vi "mWmotor_Main_calib.vi"() -> ()   [LabVIEW 2019]
uses:
  SubVI/Automatic mode/Controller decision.ctl
  SubVI/Motor Controller/Motor Class/Motor.lvclass
  SubVI/Beam/Beam.lvclass
  SubVI/Automation/Automation.lvclass
  SubVI/Simulation/Signaller/Signaller.lvclass
panel:
  out "Intensity Found":bool
  out "Last spill Intensity \n(protons)":dbl format="%#_6e"
  in  "Reset the counter":bool
  in  "Pause  accumulation":bool
  out "Spil Counter":dbl
  out "Accumulated Intensity (protons)":dbl format="%#_6e"
  out "Spill ID":dbl format="%#_6f"
  out "Current Frequencuy  (GHz)\n(Mapped)":dbl format="%_6g"
  out "EIP Frequency (GHz)":dbl format="%#_7g"
  out "Current possition (rev)":dbl
  in  "Move to frequecy":bool
  in  "Set possition (rev)":dbl=0.36 min=0.0 max=4.1
  in  "Degrees":dbl=0.36 min=0.36
  in  "CCW":bool
  in  "CW":bool
  in  "stop motor":bool
  in  "Set Freq (GHz)":dbl=140.0 min=140.0 max=141.9
  out "Upper (GHz)":dbl
  out "Lower (GHz)":dbl
  in  "Range(MHz)":dbl=10.0
  in  "Center Frequency(GHz)":dbl=140.2
  in  "Seek Function":enum16{"Rate based", "Ploarization(avg) based"}(ring)
  out "Motor Action":T1
  out "Has all samples":bool
  in  "Automatic step size (rev)":dbl=0.001
  in  "Seek type":enum32{"Seek Positive", "Seek Negative"}(radio)
  in  "Start Auto control":bool
  in  "Bypass Freq check":bool
  out "Gradients":dbl[](array[numeric])
  out "Recovery sequence":string
  in  "Recovery loop stop":bool
  in  "Recovery":bool
  out "Temp alarms":bool
  in  "Start Recovery":bool
  in  "Record Data":bool=TRUE
  in  "Warning Sound":bool
  out "EIO Temp":string
  out "chart_temp 2":waveform(dbl)[](graph)=[{"t0"=timestamp(3772890114.31303 s since 1904-01-01), "dt"=1.0, "Y"=[0.8687935985565186]}, {"t0"=timestamp(3772890114.31303 s since 1904-01-01), "dt"=1.0, "Y"=[86.87935985565186]}, {"t0"=timestamp(3772890114.31303 s since 1904-01-01), "dt"=1.0, "Y"=[30.48853325313992]}, {"t0"=timestamp(3772890114.31303 s since 1904-01-01), "dt"=1.0, "Y"=[303.6385332531399]}] caption="EIO temperatures"
  out "T_array":dbl[](array[numeric])
  out "Accumilated dose":waveform(dbl)[](graph)=[{"t0"=timestamp(3772890114.31303 s since 1904-01-01), "dt"=1.0, "Y"=[0.8687935985565186]}, {"t0"=timestamp(3772890114.31303 s since 1904-01-01), "dt"=1.0, "Y"=[86.87935985565186]}, {"t0"=timestamp(3772890114.31303 s since 1904-01-01), "dt"=1.0, "Y"=[30.48853325313992]}, {"t0"=timestamp(3772890114.31303 s since 1904-01-01), "dt"=1.0, "Y"=[303.6385332531399]}]
  out "Calibration run flag":bool
  out "New data point":bool
  out "EIPFRQ":waveform(dbl)[](graph)=[{"t0"=timestamp(3772890114.31303 s since 1904-01-01), "dt"=1.0, "Y"=[0.8687935985565186]}, {"t0"=timestamp(3772890114.31303 s since 1904-01-01), "dt"=1.0, "Y"=[86.87935985565186]}, {"t0"=timestamp(3772890114.31303 s since 1904-01-01), "dt"=1.0, "Y"=[30.48853325313992]}, {"t0"=timestamp(3772890114.31303 s since 1904-01-01), "dt"=1.0, "Y"=[303.6385332531399]}]
  out "Simulated Eventnum":i64
  out "Simulated polarization":dbl
  in  "Launch simulation":bool
  in  "Polarization data source":enum32{"NMR", "SIM"}(radio)
  out "EIO Temp reading":bool
  out "Motor alarm":bool
  out "NMR data issue":bool
  out "Loop Running":bool
  in  "NMR IP":string="192.168.24.191"
  in  "EIP":refnum<visa-resource-name>="GPIB0::5::INSTR"
  in  "ADC Port":refnum<visa-resource-name>="COM4"
  in  "stop VI":bool
  in  "Motor Port":refnum<visa-resource-name>="COM3"
  out "Current motor possition (Revolutions)":dbl(knob) caption="Current Angle" scale=0.0..4.1
  out "CCW":bool caption="CCW Limit"
  out "CW":bool caption="CW Limit"
  out "ADC Count":i32(slide) scale=0.0..32768.0
  out "ADC Count":i32
  out "Motor Running":bool
  out "Polarization":dbl format="%#_3f"
  out "Eventnum":i64
  out "Polarization Chart":waveform(dbl)[](graph)=[{"t0"=timestamp(3772890114.31303 s since 1904-01-01), "dt"=1.0, "Y"=[0.8687935985565186]}, {"t0"=timestamp(3772890114.31303 s since 1904-01-01), "dt"=1.0, "Y"=[86.87935985565186]}, {"t0"=timestamp(3772890114.31303 s since 1904-01-01), "dt"=1.0, "Y"=[30.48853325313992]}, {"t0"=timestamp(3772890114.31303 s since 1904-01-01), "dt"=1.0, "Y"=[303.6385332531399]}]
  in  "Calibration panel":bool
  in  "Calibration panel":enum32{"Page 1", "Page 2"}(tab)
  out "Lower Frequency":dbl
  out "Lower  possition":dbl
  in  "R_lower":bool
  out "New Intercept":dbl=138.611
  out "New Slope":dbl=0.864
  in  "Use_para":bool
  out "Upper  possition":dbl
  in  "cal_para":bool
  out "Upper Frequecy":dbl
  in  "R_upper":bool
  out "Intercept":dbl
  out "Slope":dbl
  in  "Set_motor":bool
  in  "File Path Control":path=path "C:/Users/ptgroup/Desktop/github/Microwave-motor-control/config.ini"
  out "Speed  (rev/s)":dbl
  in  "File Name":string
  out "Frequency (GHz)":dbl
  out "Possition (Rev)":dbl format="%_4g"
  out "New data  saved":bool
  out "Recording":bool
  in  "Stop calibration":bool
  in  "Move direction":enum32{"CCW", "CW"}(radio)
  in  "Start calibration":bool
  in  "Step size (rev)":dbl
  out "Estimated Possition":dbl
  out "error out":errorcluster
  # "Warnings"
  # "Manual Motor Control"
  # "Beam information"
  # "Auto control   Setup"
  # "Auto control   Parameters"
  # "Communication  Setup"
  # "Current motor possition (Rev)"
  # "Calibration Panel"
  # "Calibration panel"
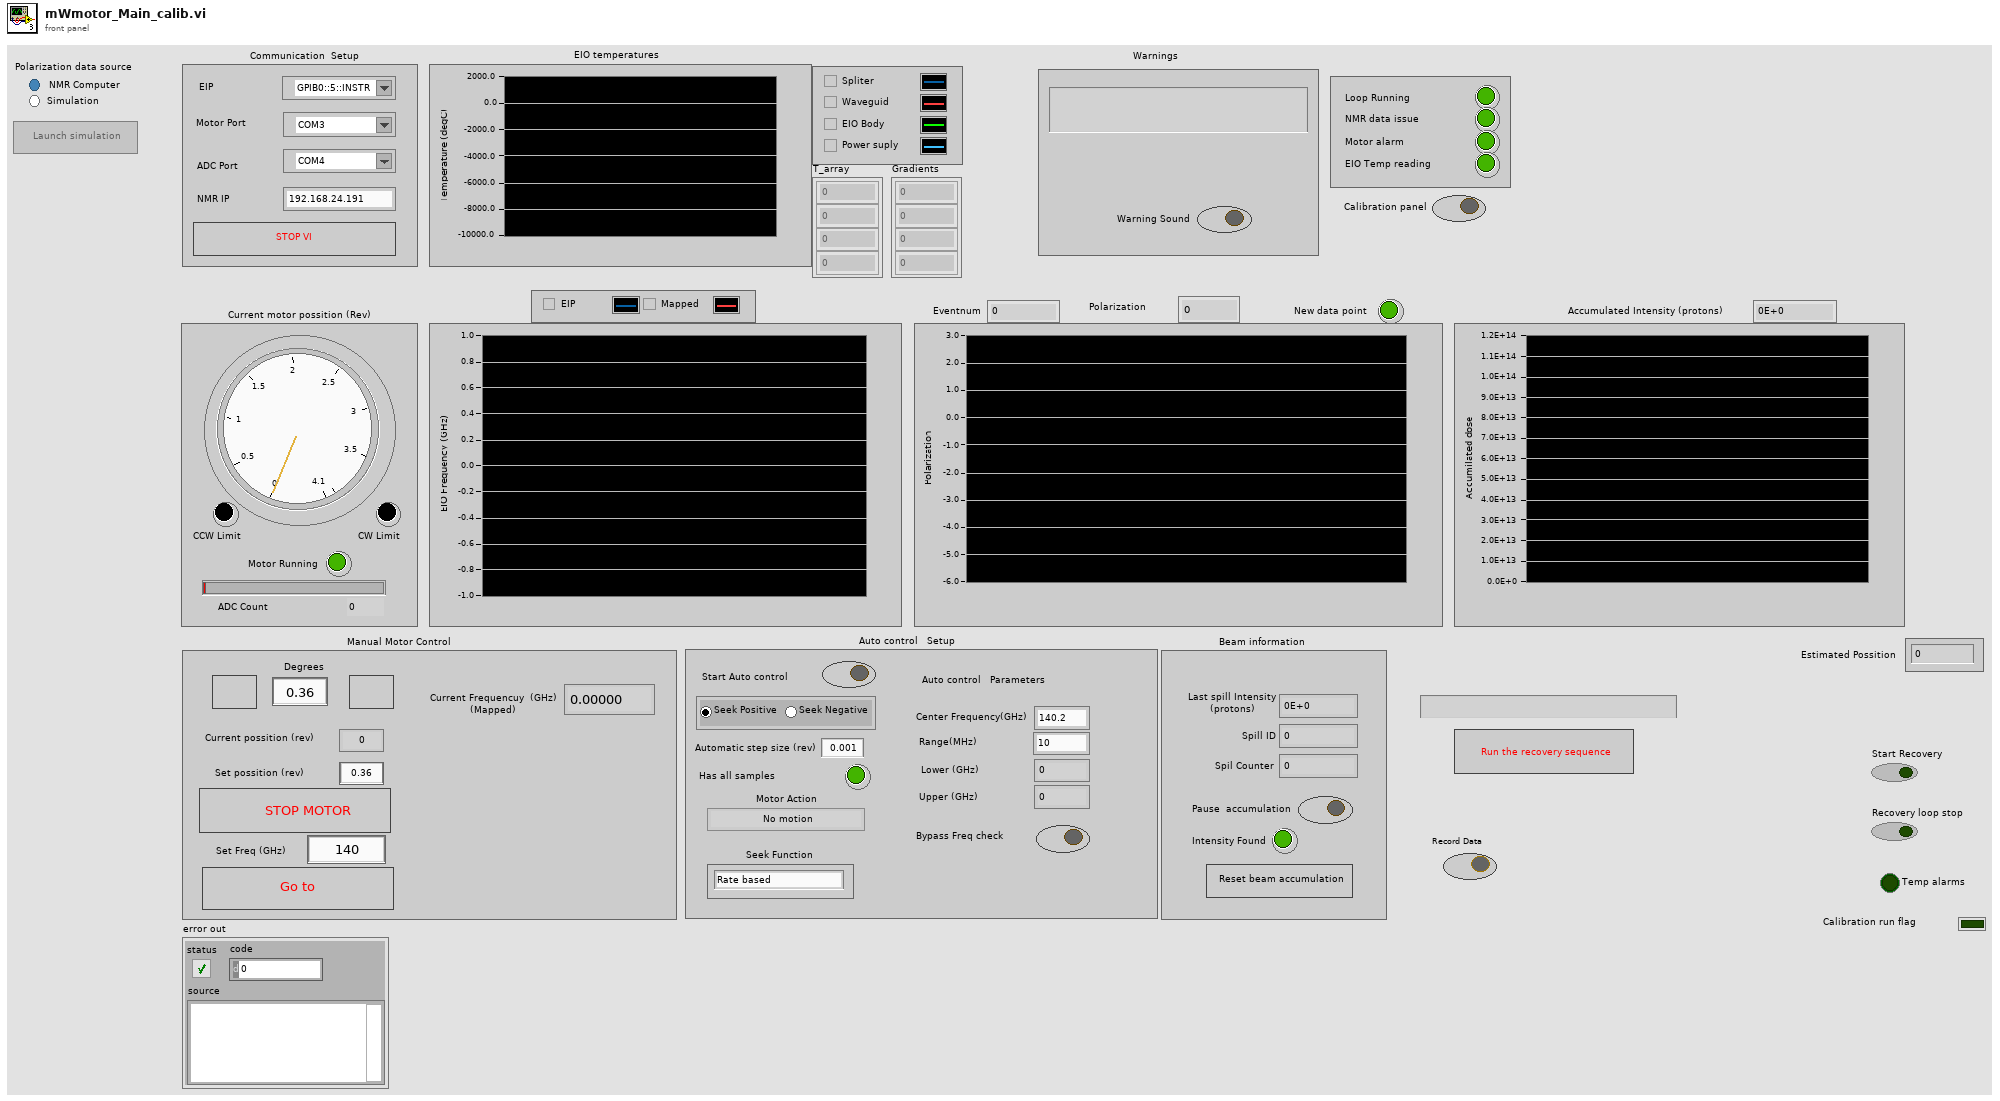
[diagram p1: front panel]
types:
  T1 = typedef "Controller decision.ctl" = enum16{"No motion", "Switch direction", "Keep current direction"}
  T2 = enum8{"Enabled", "Disabled", "Disabled and Grayed Out"}
  T3 = typedef "Sound Output Task ID.ctl" = u32
  T4 = enum32{"Bad", "Idle", "Run top level", "Running"}
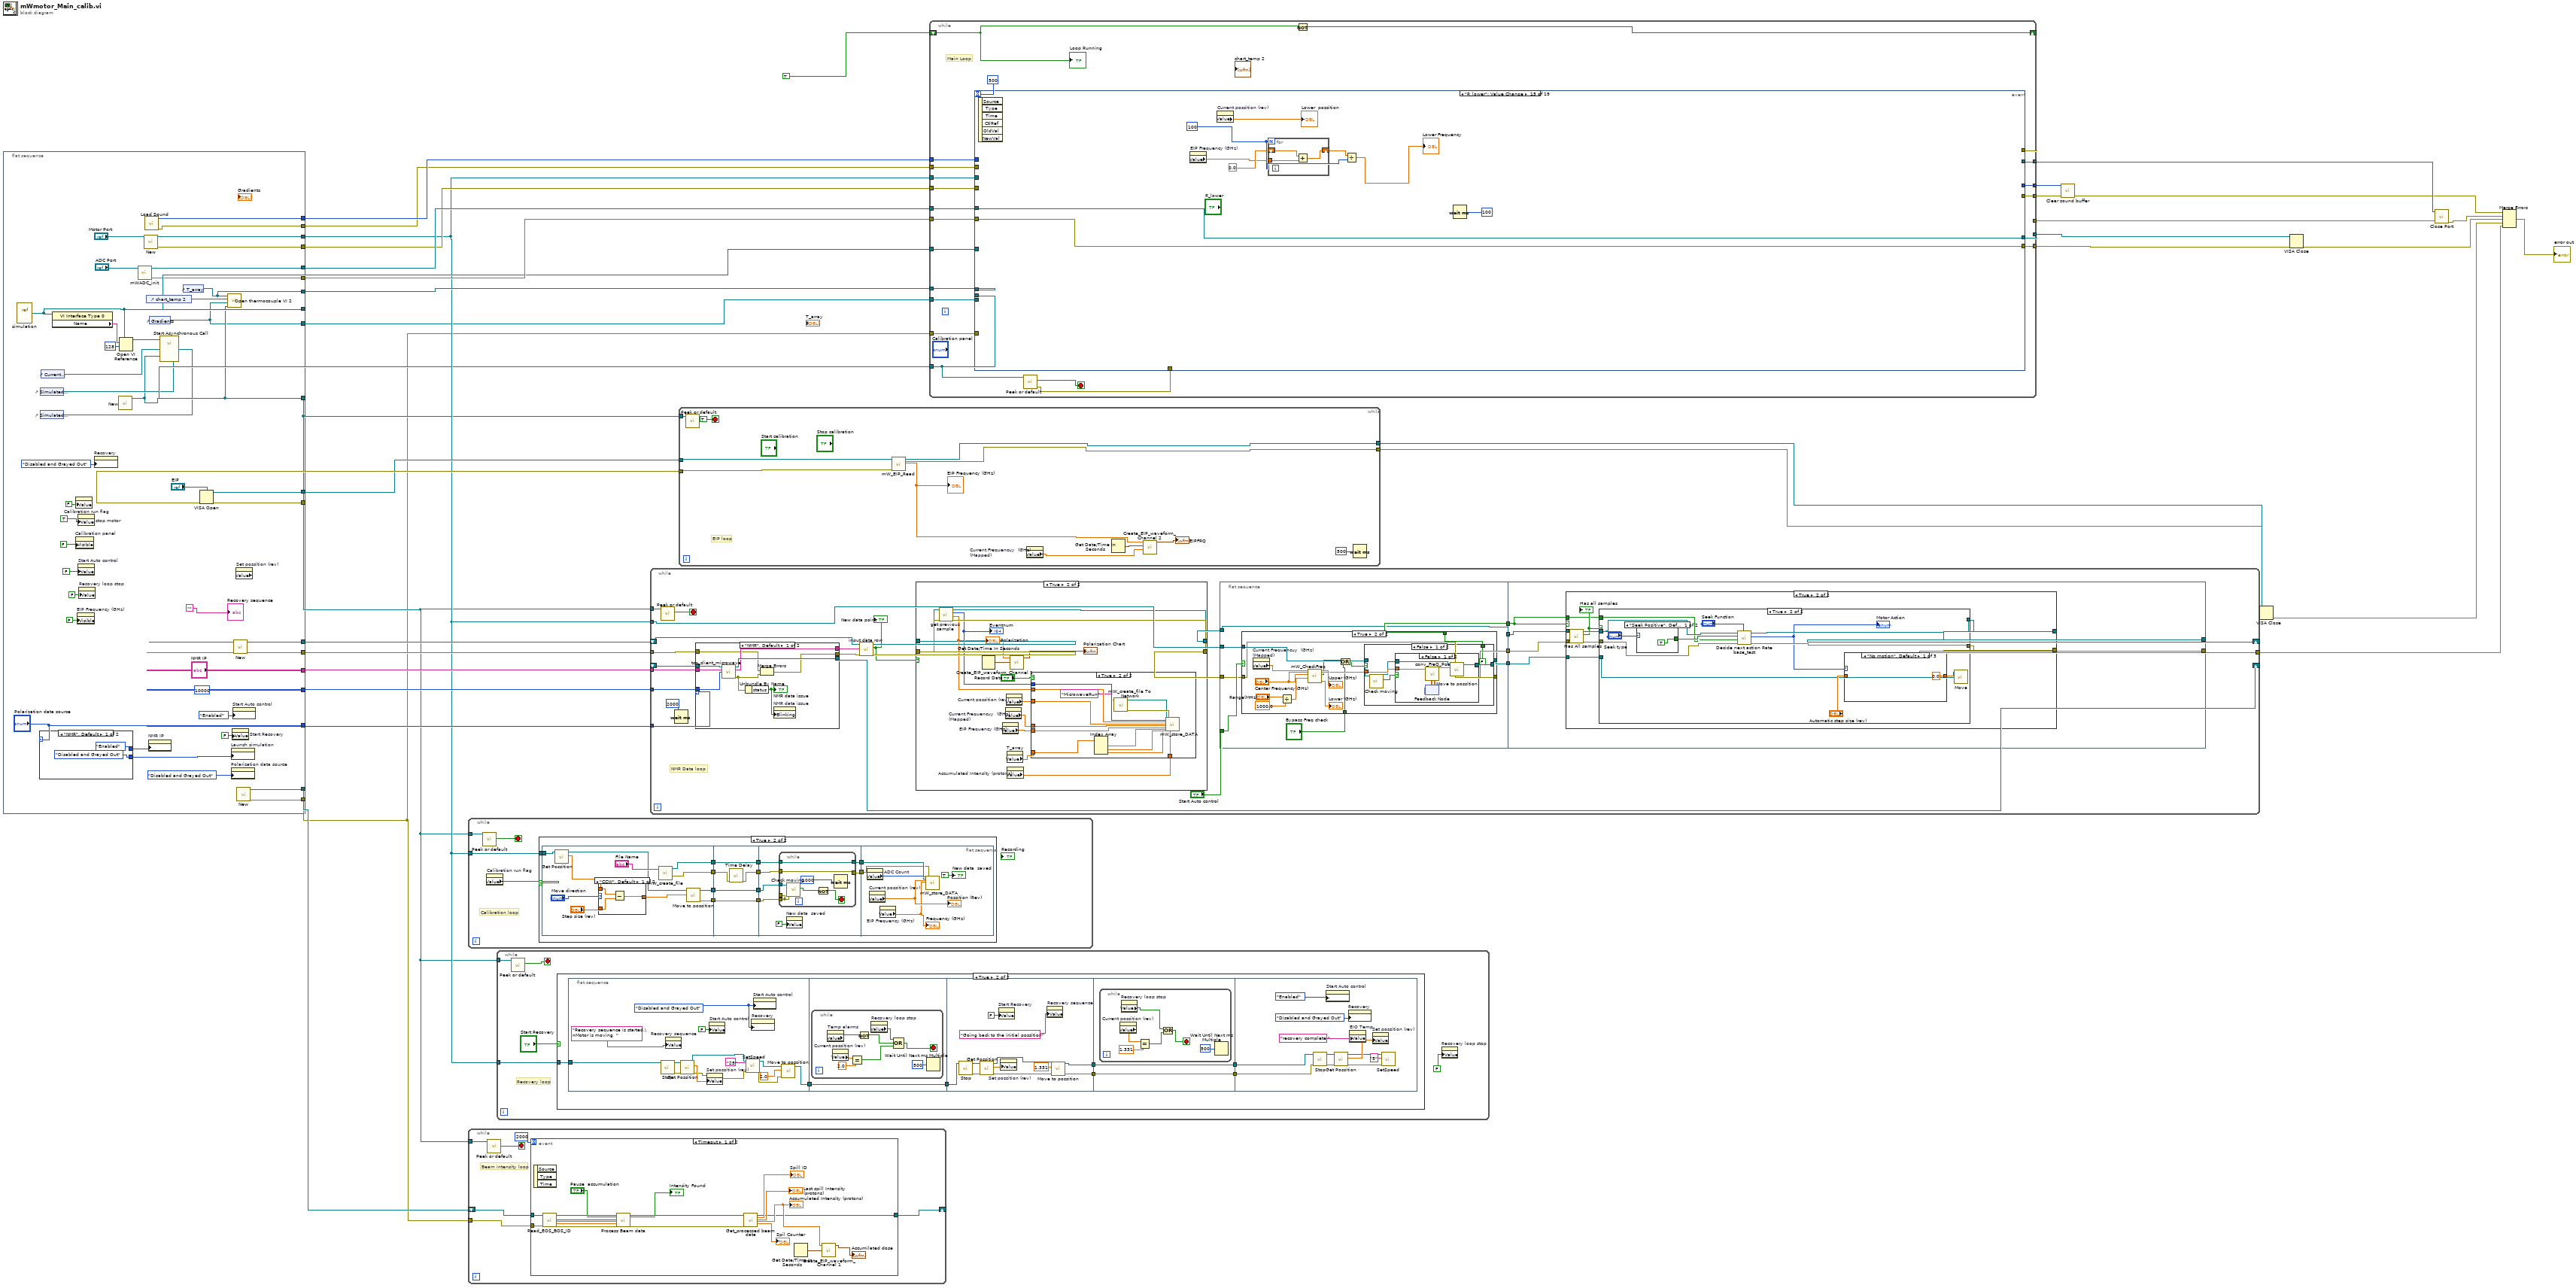
[diagram p0: block diagram]
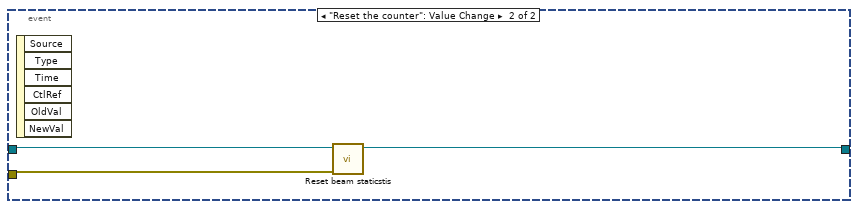
[diagram p2: hidden frame]
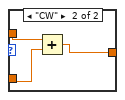
[diagram p5: hidden frame]
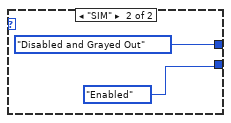
[diagram p6: hidden frame]
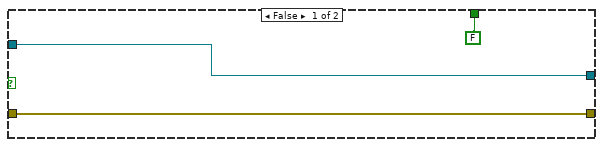
[diagram p7: hidden frame]
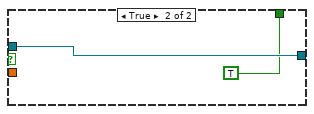
[diagram p9: hidden frame]
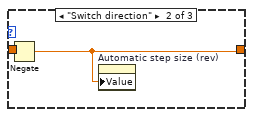
[diagram p12: hidden frame]
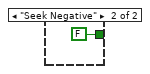
[diagram p14: hidden frame]
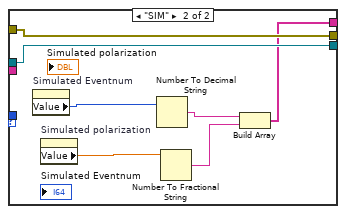
[diagram p17: hidden frame]
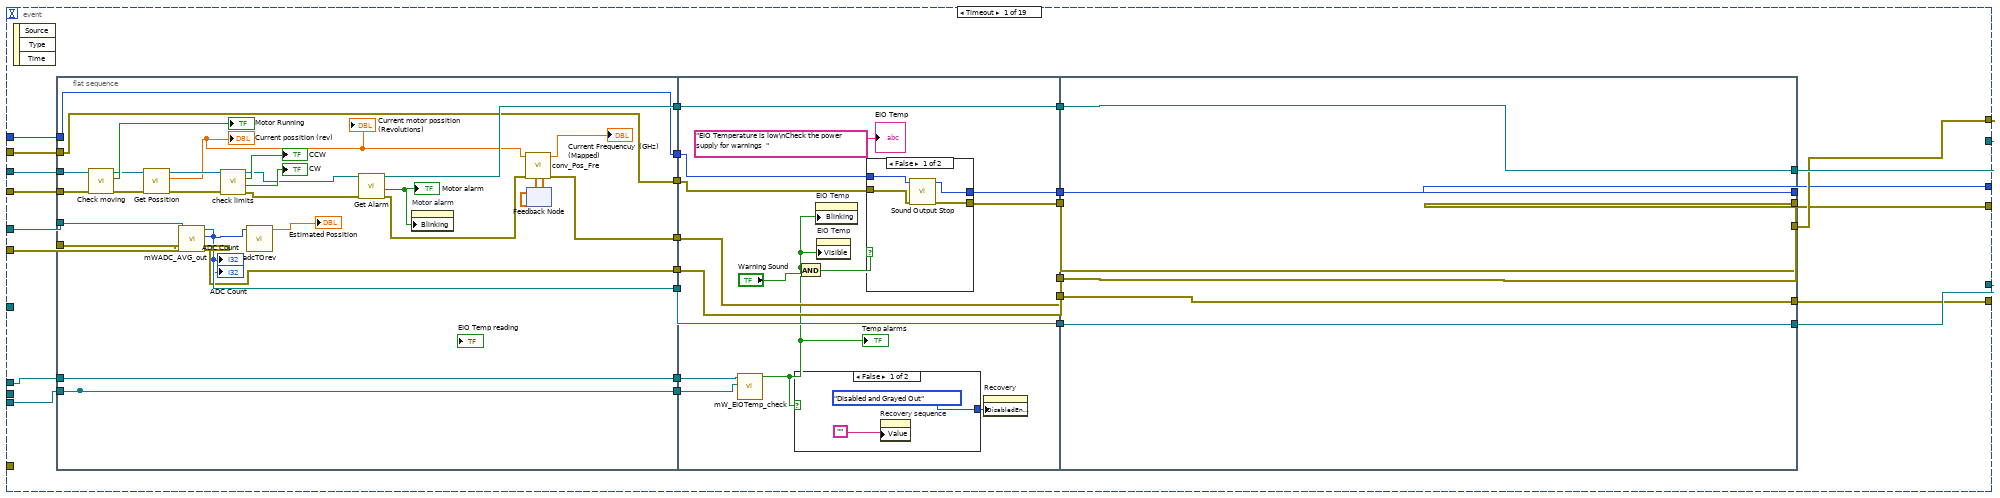
[diagram p18: hidden frame]
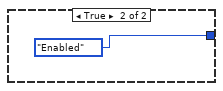
[diagram p19: hidden frame]
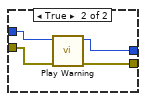
[diagram p20: hidden frame]
diagram:
  n1 = flat-sequence {
    tunnel: [w75] -> w33
    tunnel: [w74] -> w30
    tunnel: [w73] -> w27
    tunnel: [w72] -> w26
    tunnel: [w68] -> w5
    tunnel: [w67] -> w23
    tunnel: [u16 10000 ("port")] -> w18
    tunnel: [w65] -> w17
    tunnel: [w64] -> w16
    tunnel: ["NMR IP"] -> w15
    tunnel: [w60] -> w13
    tunnel: [w47] -> w3
    tunnel: ["Polarization data source"] -> w12
    tunnel: [w46] -> w11
    tunnel: [w45] -> w10
    tunnel: [w44] -> w9
    tunnel: [w38] -> w4
    tunnel: [w37] -> w2
    tunnel: [w36] -> w1
    frame #0 {
      n2 = vi-ref "simulation.vi"() -> (w60:refnum<vi>)
      n3 = case shown="\"NMR\", Default" "Polarization data source" {
        tunnel: [T2."Disabled and Grayed Out" ("Disabled") T2."Enabled" ("Disabled")] -> w54
        tunnel: [T2."Enabled" ("Disabled") T2."Disabled and Grayed Out" ("Disabled")] -> w52
        frame "NMR", Default {
        }
        frame "SIM" {
        }
      }
      n4 = control-ref of="Simulated Eventnum"() -> (w56:refnum<vi>)
      n5 = control-ref of="Simulated polarization"() -> (w57:refnum<vi>)
      n6 = control-ref of="Current Frequencuy  (GHz)\n(Mapped)"() -> (w58:refnum<vi>)
      n7 = property class="VI Interface Type 0"(reference=w60) -> ("Name"=w62:string)  [unwired: 1 in, 2 out]
      n8 = property on="Calibration panel" class="TabCtl (strict)"("Visible"=FALSE) -> ()  [unwired: 2 in, 2 out]
      n9 = property on="Calibration run flag" class="Bool (strict)"("Value"=FALSE ("Calibration run flag")) -> ()  [unwired: 2 in, 2 out]
      n10 = property on="EIP Frequency (GHz)" class="DigNum (strict)"("Visible"=FALSE) -> ()  [unwired: 2 in, 2 out]
      n11 = property on="stop motor" class="Bool (strict)"("Value"=TRUE ("Value (Signaling)")) -> ()  [unwired: 2 in, 2 out]
      n12 = property on="Start Auto control" class="Bool (strict)"("Value"=FALSE ("Start Auto control")) -> ()  [unwired: 2 in, 2 out]
      n13 = property on="Recovery loop stop" class="Bool (strict)"("Value"=FALSE ("Recovery loop stop")) -> ()  [unwired: 2 in, 2 out]
      n14 = property on="Recovery" class="Bool (strict)"("DisabledEnum"=T2."Disabled and Grayed Out" ("Disabled")) -> ()  [unwired: 2 in, 2 out]
      n15 = call "New.vi"() -> ("Signaller out"=w47:refnum<class "Signaller.lvclass">)  [unwired: 11 in]
      n16 = Open VI Reference(type specifier VI Refnum (for type only)=w60, vi path=w62, options=128) -> (vi reference=w59:refnum<vi>)  [unwired: 3 in, 1 out]
      n17 = call "mWADC_init.vi"("mWADC_Port"="ADC Port") -> ("error out"=w74:errorcluster, "reference out"=w75:refnum<visa-resource-name>)  [unwired: 9 in]
      n18 = call "New.vi"("VISA resource name"="Motor Port") -> ("error out"=w67:errorcluster, "Motor out"=w68:refnum<class "Motor.lvclass">)  [unwired: 9 in]
      n19 = call "Load Sound.vi"() -> ("error out"=w44:errorcluster, "task ID out"=w45:T3)  [unwired: 10 in]
      n20 = control-ref of="chart_temp 2"() -> (w48:refnum<vi>)
      n21 = property on="NMR IP" class="Str"("DisabledEnum"=w52) -> ()  [unwired: 2 in, 2 out]
      n22 = control-ref of="Gradients"() -> (w38:refnum<vi>)
      n23 = call-by-ref "Start Asynchronous Call"(reference=w59, "Eventnum refnum"=w56, "Polarization refnum"=w57, "Stop signaller"=w47, "Frequency refnum"=w58) -> ()  [unwired: 1 in, 2 out]
      n24 = control-ref of="T_array"() -> (w46:refnum<vi>)
      n25 = VISA Open(VISA resource name="EIP") -> (VISA resource name=w72:refnum<visa-resource-name>, error out=w73:errorcluster)  [unwired: 4 in]
      n26 = call "Open thermocouple VI 2.vi"("Signaller in"=w47, "Gradients"=w38, "chart_temp ref"=w48, "Temperaturs"=w46) -> ()  [unwired: 8 in]
      n27 = property on="Launch simulation" class="Bool"("DisabledEnum"=w54) -> ()  [unwired: 2 in, 2 out]
      n28 = property on="Polarization data source" class="RadioBtnsControl (strict)"("DisabledEnum"=T2."Disabled and Grayed Out" ("Disabled")) -> ()  [unwired: 2 in, 2 out]
      n29 = property on="Start Recovery" class="Bool (strict)"("Value"=FALSE ("Start Recovery")) -> ()  [unwired: 2 in, 2 out]
      n30 = property on="Start Auto control" class="Bool (strict)"("DisabledEnum"=T2."Enabled" ("Disabled")) -> ()  [unwired: 2 in, 2 out]
      n31 = call "New.vi"() -> ("error out"=w64:errorcluster, "Automation out"=w65:refnum<class "Automation.lvclass">)  [unwired: 10 in]
      n32 = property on="Set possition (rev)" class="DigNum (strict)" props=["Value"]() -> ()  [unwired: 2 in, 3 out]
      n33 = call "New.vi"() -> ("error out"=w36:errorcluster, "Beam out"=w37:refnum<class "Beam.lvclass">)  [unwired: 10 in]
      "Recovery sequence" <- ""
    }
  }
  n34 = while {
    tunnel: w3 -> [w84]
    tunnel: w5 -> [w82]
    stop <- w81 stop-if-true
    # "Calibration loop"
    n35 = call "Peek or default.vi"("Signaller in"=w84) -> ("Has signal?"=w81:bool)  [unwired: 8 in, 2 out]
    n36 = property on="Calibration run flag" class="Bool (strict)"() -> ("Value"=w83:bool)  [unwired: 2 in, 2 out]
    n37 = case shown="True" w83 {
      tunnel: w82 -> [_ w89]
      frame False {
      }
      frame True {
        n38 = flat-sequence {
          tunnel: [w106] -> w93
          tunnel: [w105] -> w91
          tunnel: w89 -> [w100]
          tunnel: [w97] -> w88
          tunnel: [w96] -> w85
          tunnel: w93 -> [w116]
          tunnel: [w115] -> w92
          tunnel: w91 -> [w117]
          tunnel: [w117] -> w90
          tunnel: w88 -> [w114]
          tunnel: [w114] -> w87
          tunnel: [w113] -> w86
          tunnel: w85 -> [w113]
          tunnel: [w123] -> w95
          tunnel: w92 -> [w124]
          tunnel: w90 -> [w121]
          tunnel: [w122] -> w94
          tunnel: w87 -> [w119]
          tunnel: w86 -> [w120]
          tunnel: w95 -> [w132]
          tunnel: w94 -> [w136]
          frame #0 {
            n39 = call "Get Possition.vi"("Motor in"=w100) -> ("Revolutions"=w101:dbl, "Motor out"=w98:refnum<class "Motor.lvclass">)  [unwired: 8 in, 1 out]
            n40 = case shown="\"CCW\", Default" "Move direction" {
              tunnel: [w107 w112] -> w99
              tunnel: "Step size (rev)" -> [w108 w111]
              tunnel: w101 -> [w109 w110]
              frame "CCW", Default {
                n41 = Subtract(x=w109, y=w108) -> (x-y=w107:dbl)
              }
              frame "CW" {
                n42 = Add(x=w110, y=w111) -> (x+y=w112:dbl)
              }
            }
            n43 = call "mW_create_file.vi"("File Name"="File Name") -> ("error out"=w106:errorcluster, "dup path"=w105:path)  [unwired: 9 in]
            n44 = call "Move to possition.vi"("absolute possition(rev)"=w99, "Motor in"=w98) -> ("error out"=w97:errorcluster, "Motor out"=w96:refnum<class "Motor.lvclass">)  [unwired: 8 in]
          }
          frame #1 {
            n45 = call "Time Delay"("error in (no error)"=w116) -> ("error out"=w115:errorcluster)  [unwired: 10 in]
          }
          frame #2 {
            n46 = while {
              tunnel: [w130] -> w123
              tunnel: w124 -> [w130]
              tunnel: [w129] -> w122
              tunnel: w121 -> [w129]
              tunnel: w120 -> [w127]
              tunnel: w119 -> [w125]
              tunnel: [w125] -> _
              stop <- w131 stop-if-true
              n47 = call "Check moving.vi"("error in (no error)"=w125, "Motor in"=w127) -> ("IS Move"=w128:bool)  [unwired: 7 in, 2 out]
              n48 = Not(x=w128) -> (.not. x?=w131:bool)
              n49 = Wait (ms)(milliseconds to wait=u32 1000) -> ()  [unwired: 1 out]
            }
            n50 = property on="New data  saved" class="Bool (strict)"("Value"=FALSE ("New data  saved")) -> ()  [unwired: 2 in, 2 out]
          }
          frame #3 {
            n51 = property on="ADC Count" class="DigNum (strict)"() -> ("Value"=w135:i32)  [unwired: 2 in, 2 out]
            n52 = property on="Current possition (rev)" class="DigNum (strict)"() -> ("Value"=w134:dbl)  [unwired: 2 in, 2 out]
            "Possition (Rev)" <- w134
            n53 = property on="EIP Frequency (GHz)" class="DigNum (strict)"() -> ("Value"=w133:dbl)  [unwired: 2 in, 2 out]
            "Frequency (GHz)" <- w133
            n54 = call "mW_store_DATA.vi"("file path (dialog if empty)"=w136, "col1"=w135, "col2"=w134, "col3"=w133, "error in (no error)"=w132) -> ()  [unwired: 22 in, 1 out]
            "New data  saved" <- TRUE ("New data  saved")
          }
        }
      }
    }
  }
  n55 = while {
    tunnel: w3 -> [w143]
    tunnel: w1 -> [w141]
    shift-right: [w140] -> _
    shift-left: w2 -> [w142]
    stop <- w138 stop-if-true
    # "Beam intensity loop"
    n56 = call "Peek or default.vi"("Signaller in"=w143) -> ("Has signal?"=w138:bool)  [unwired: 8 in, 2 out]
    n57 = event shown="[0] Timeout" {
      selector: _ -> [_ _]
      dyn-events: _ -> [_ _]
      timeout: 2000 -> [_ _]
      tunnel: w142 -> [w161 w164]
      tunnel: w141 -> [w160 w163]
      tunnel: [w153 w162] -> w140
      event Timeout {
        n58 = event-data() -> ()  [unwired: 1 in, 3 out]
        n59 = call-dynamic "Read_EOS_BOS_ID.vi"("Beam in"=w161, "error in (no error)"=w160) -> ("Beam out"=w147:refnum<class "Beam.lvclass">, "Spill ID"=w150:i32, "BOS Time"=w149:dbl, "EOS Time"=w148:dbl, "error out"=w152:errorcluster)  [unwired: 8 in, 1 out]
        n60 = call "Process Beam data.vi"("Beam in"=w147, "Pause"="Pause  accumulation", "Spill ID"=w150, "BOS"=w149, "EOS"=w148, "error in (no error)"=w152) -> ("Beam out"=w146:refnum<class "Beam.lvclass">, "Intensity Found"=→"Intensity Found":bool, "error out"=w151:errorcluster)  [unwired: 11 in]
        n61 = call "Get_processed beam data.vi"("Beam in"=w146, "error in (no error)"=w151) -> ("Beam out"=w153:refnum<class "Beam.lvclass">, "Spill ID"=→"Spill ID":dbl, "Recent spill Intensity"=→"Last spill Intensity \n(protons)":dbl, "Acumilated Intensity"=w156:dbl, "Spil Counter"=→"Spil Counter":dbl)  [unwired: 12 in, 1 out]
        "Accumulated Intensity (protons)" <- w156
        n62 = Get Date/Time In Seconds() -> (seconds since 1Jan1904=w157:timestamp)
        n63 = call "Create_EIP_waveform_Channel 1.vi"("time"=w157, "Channel 1"=w156) -> ("waveform_array"=→"Accumilated dose":waveform(dbl)[])  [unwired: 9 in]
      }
      event "Reset the counter": Value Change {
        n64 = event-data() -> ()  [unwired: 1 in, 6 out]
        n65 = call "Reset beam staticstis.vi"("error in (no error)"=w163, "Beam in"=w164) -> ("Beam out"=w162:refnum<class "Beam.lvclass">)  [unwired: 8 in, 1 out]
      }
    }
  }
  n66 = while {
    tunnel: w3 -> [w169]
    tunnel: w5 -> [w167]
    stop <- w165 stop-if-true
    # "Recovery loop"
    n67 = call "Peek or default.vi"("Signaller in"=w169) -> ("Has signal?"=w165:bool)  [unwired: 8 in, 2 out]
    n68 = case shown="True" "Start Recovery" {
      tunnel: w167 -> [_ w176]
      frame False {
      }
      frame True {
        n69 = flat-sequence {
          tunnel: w176 -> [w187]
          tunnel: [w184] -> w175
          tunnel: w175 -> [w192]
          tunnel: [w192] -> w174
          tunnel: w174 -> [w209]
          tunnel: [w203] -> w172
          tunnel: [w202] -> w170
          tunnel: [w213] -> w173
          tunnel: w172 -> [w213]
          tunnel: [w212] -> w171
          tunnel: w170 -> [w212]
          tunnel: w173 -> [w227]
          tunnel: w171 -> [w226]
          frame #0 {
            w182 = T2."Disabled and Grayed Out" ("Disabled")
            n70 = call "Stop.vi"("Motor in"=w187) -> ("error out"=w190:errorcluster, "Motor out"=w189:refnum<class "Motor.lvclass">)  [unwired: 9 in]
            n71 = property on="Recovery sequence" class="Str"("Value"="Recovery sequence is started.\nMotor is moving  " ("EIO Temp")) -> ()  [unwired: 2 in, 2 out]
            n72 = call "Get Possition.vi"("error in (no error)"=w190, "Motor in"=w189) -> ("error out"=w185:errorcluster, "Revolutions"=w188:dbl, "Motor out"=w181:refnum<class "Motor.lvclass">)  [unwired: 7 in]
            n73 = property on="Set possition (rev)" class="DigNum (strict)"(error in=w185, "Value"=w188) -> (error out=w179:errorcluster)  [unwired: 1 in, 1 out]
            n74 = property on="Start Auto control" class="Bool (strict)"("Value"=FALSE ("Start Auto control")) -> ()  [unwired: 2 in, 2 out]
            n75 = call "SetSpeed.vi"("error in (no error)"=w179, "Speed"="25", "Motor in"=w181) -> ("error out"=w178:errorcluster, "Motor out"=w180:refnum<class "Motor.lvclass">)  [unwired: 7 in]
            n76 = property on="Recovery" class="Bool (strict)"("DisabledEnum"=w182) -> ()  [unwired: 2 in, 2 out]
            n77 = property on="Start Auto control" class="Bool (strict)"("DisabledEnum"=w182) -> ()  [unwired: 2 in, 2 out]
            n78 = call "Move to possition.vi"("error in (no error)"=w178, "absolute possition(rev)"=2.0, "Motor in"=w180) -> ("Motor out"=w184:refnum<class "Motor.lvclass">)  [unwired: 7 in, 1 out]
          }
          frame #1 {
            n79 = while {
              stop <- w193 stop-if-true
              n80 = property on="Temp alarms" class="Bool (strict)"() -> ("Value"=w200:bool)  [unwired: 2 in, 2 out]
              n81 = property on="Current possition (rev)" class="DigNum (strict)"() -> ("Value"=w198:dbl)  [unwired: 2 in, 2 out]
              n82 = Equal?(x=w198, y=2.0) -> (x = y?=w196:bool)
              n83 = Not(x=w200) -> (.not. x?=w195:bool)
              n84 = property on="Recovery loop stop" class="Bool (strict)"() -> ("Value"=w194:bool)  [unwired: 2 in, 2 out]
              n85 = Compound Arithmetic op=OR(w194, w195, w196) -> (w193:bool)
              n86 = Wait Until Next ms Multiple(millisecond multiple=u32 500) -> ()  [unwired: 1 out]
            }
          }
          frame #2 {
            n87 = call "Stop.vi"("Motor in"=w209) -> ("error out"=w211:errorcluster, "Motor out"=w210:refnum<class "Motor.lvclass">)  [unwired: 9 in]
            n88 = call "Get Possition.vi"("error in (no error)"=w211, "Motor in"=w210) -> ("error out"=w205:errorcluster, "Revolutions"=w208:dbl, "Motor out"=w206:refnum<class "Motor.lvclass">)  [unwired: 7 in]
            n89 = property on="Start Recovery" class="Bool (strict)"("Value"=FALSE ("Start Recovery")) -> ()  [unwired: 2 in, 2 out]
            n90 = property on="Set possition (rev)" class="DigNum (strict)"("Value"=w208) -> ()  [unwired: 2 in, 2 out]
            n91 = property on="Recovery sequence" class="Str"("Value"="Going back to the initial possition" ("EIO Temp")) -> ()  [unwired: 2 in, 2 out]
            n92 = call "Move to possition.vi"("error in (no error)"=w205, "absolute possition(rev)"=1.331, "Motor in"=w206) -> ("error out"=w203:errorcluster, "Motor out"=w202:refnum<class "Motor.lvclass">)  [unwired: 7 in]
          }
          frame #3 {
            n93 = while {
              stop <- w216 stop-if-true
              n94 = property on="Current possition (rev)" class="DigNum (strict)"() -> ("Value"=w218:dbl)  [unwired: 2 in, 2 out]
              n95 = property on="Recovery loop stop" class="Bool (strict)"() -> ("Value"=w214:bool)  [unwired: 2 in, 2 out]
              n96 = Equal?(x=w218, y=1.331) -> (x = y?=w215:bool)
              n97 = Or(x=w214, y=w215) -> (x .or. y?=w216:bool)
              n98 = Wait Until Next ms Multiple(millisecond multiple=u32 500) -> ()  [unwired: 1 out]
            }
          }
          frame #4 {
            n99 = call "Stop.vi"("error in (no error)"=w227, "Motor in"=w226) -> ("error out"=w228:errorcluster, "Motor out"=w229:refnum<class "Motor.lvclass">)  [unwired: 8 in]
            n100 = property on="Start Auto control" class="Bool (strict)"("DisabledEnum"=T2."Enabled" ("Disabled")) -> ()  [unwired: 2 in, 2 out]
            n101 = call "Get Possition.vi"("error in (no error)"=w228, "Motor in"=w229) -> ("error out"=w221:errorcluster, "Revolutions"=w230:dbl, "Motor out"=w222:refnum<class "Motor.lvclass">)  [unwired: 7 in]
            n102 = property on="Recovery" class="Bool (strict)"("DisabledEnum"=T2."Disabled and Grayed Out" ("Disabled")) -> ()  [unwired: 2 in, 2 out]
            n103 = property on="EIO Temp" class="Str"("Value"="recovery complete " ("EIO Temp")) -> ()  [unwired: 2 in, 2 out]
            n104 = property on="Set possition (rev)" class="DigNum (strict)"("Value"=w230) -> ()  [unwired: 2 in, 2 out]
            n105 = call "SetSpeed.vi"("error in (no error)"=w221, "Speed"="5", "Motor in"=w222) -> ()  [unwired: 7 in, 2 out]
          }
        }
      }
    }
    n106 = property on="Recovery loop stop" class="Bool (strict)"("Value"=FALSE ("Recovery loop stop")) -> ()  [unwired: 2 in, 2 out]
  }
  n107 = while {
    tunnel: w15 -> [w255]
    tunnel: w18 -> [w254]
    shift-right: [w252] -> _
    shift-left: _ -> [w253]
    tunnel: w16 -> [w245]
    shift-right: [w239] -> _
    shift-left: w17 -> [w249]
    tunnel: [w238] -> w14
    tunnel: w3 -> [w244]
    tunnel: w12 -> [w243]
    tunnel: w5 -> [w237]
    stop <- w231 stop-if-true
    # "NMR Data loop"
    n108 = call "Peek or default.vi"("Signaller in"=w244) -> ("Has signal?"=w231:bool)  [unwired: 8 in, 2 out]
    n109 = Wait (ms)(milliseconds to wait=u32 2000) -> ()  [unwired: 1 out]
    n110 = case shown="\"NMR\", Default" w243 {
      tunnel: w255 -> [w370 _]
      tunnel: w254 -> [w369 _]
      tunnel: w253 -> [w368 w376]
      tunnel: [w367 w376] -> w252
      tunnel: [w366 w374] -> w250
      tunnel: [w364 w377] -> w246
      tunnel: w245 -> [w363 w377]
      frame "NMR", Default {
        n111 = call "tcp_client_microwave.vi"("conn_id_in"=w368, "addr"=w370, "port"=w369) -> ("conn_id_out"=w367:refnum<k5>, "Raw data array"=w366:string[], "error out"=w365:errorcluster)  [unwired: 8 in, 2 out]
        n112 = Unbundle By Name(w365) -> ("status"=w362:bool)
        "NMR data issue" <- w362
        n113 = Merge Errors(w363, w365) -> (w364:errorcluster)
        n114 = property on="NMR data issue" class="Bool (strict)"("Blinking"=w362) -> ()  [unwired: 2 in, 2 out]
      }
      frame "SIM" {
        n115 = property on="Simulated Eventnum" class="DigNum (strict)"() -> ("Value"=w371:i64)  [unwired: 2 in, 2 out]
        n116 = property on="Simulated polarization" class="DigNum (strict)"() -> ("Value"=w375:dbl)  [unwired: 2 in, 2 out]
        n117 = Number To Decimal String(number=w371) -> (decimal integer string=w372:string)  [unwired: 1 in]
        n118 = Number To Fractional String(number=w375) -> (F-format string=w373:string)  [unwired: 3 in]
        n119 = Build Array(w372, w373) -> (w374:string[])
      }
    }
    n120 = call "input data row.vi"("error in (no error)"=w246, "Last row of data file"=w250, "Automation in"=w249) -> ("error out"=w248:errorcluster, "Added new data point?"=w232:bool, "Automation out"=w247:refnum<class "Automation.lvclass">)  [unwired: 4 in, 2 out]
    "New data point" <- w232
    n121 = case shown="True" w232 {
      tunnel: w248 -> [w333 w348]
      tunnel: w247 -> [w334 w347]
      tunnel: [w333 w346] -> w234
      tunnel: [w334 w345] -> w235
      frame False {
      }
      frame True {
        n122 = call "get previous sample.vi"("error in (no error)"=w348, "Automation in"=w347) -> ("error out"=w346:errorcluster, "Polarization"=w339:dbl, "Eventnum"=w340:i64, "Automation out"=w345:refnum<class "Automation.lvclass">)  [unwired: 6 in]
        "Eventnum" <- w340
        "Polarization" <- w339
        n123 = Get Date/Time In Seconds() -> (seconds since 1Jan1904=w343:timestamp)
        n124 = property on="EIP Frequency (GHz)" class="DigNum (strict)"() -> ("Value"=w336:dbl)  [unwired: 2 in, 2 out]
        n125 = property on="Current Frequencuy  (GHz)\n(Mapped)" class="DigNum (strict)"() -> ("Value"=w337:dbl)  [unwired: 2 in, 2 out]
        n126 = property on="Current possition (rev)" class="DigNum (strict)"() -> ("Value"=w338:dbl)  [unwired: 2 in, 2 out]
        n127 = property on="T_array" class="Arr (strict)"() -> ("Value"=w342:dbl[])  [unwired: 2 in, 2 out]
        n128 = property on="Accumulated Intensity (protons)" class="DigNum (strict)"() -> ("Value"=w335:dbl)  [unwired: 2 in, 2 out]
        n129 = call "Create_EIP_waveform_Channel 1.vi"("time"=w343, "Channel 1"=w339) -> ("waveform_array"=→"Polarization Chart":waveform(dbl)[])  [unwired: 9 in]
        n130 = case shown="True" "Record Data" {
          tunnel: w342 -> [_ w361]
          tunnel: w340 -> [_ w360]
          tunnel: w339 -> [_ w359]
          tunnel: w338 -> [_ w358]
          tunnel: w337 -> [_ w357]
          tunnel: w336 -> [_ w356]
          tunnel: w335 -> [_ w349]
          frame False {
          }
          frame True {
            n131 = Index Array(array=w361) -> (element #1=w355:dbl, element #2=w354:dbl, element #3=w353:dbl)  [unwired: 3 in]
            n132 = call "mW_create_file To Network.vi"("File Name"="MicrowaveRun") -> ("error out"=w352:errorcluster, "dup path"=w350:path)  [unwired: 9 in]
            n133 = call "mW_store_DATA.vi"("file path (dialog if empty)"=w350, "col1"=w360, "col2"=w359, "col3"=w358, "col4"=w357, "col5"=w356, "col6"=w355, "col7"=w354, "error in (no error)"=w352, "col8"=w353, "col9"=w349) -> ()  [unwired: 16 in, 1 out]
          }
        }
      }
    }
    n134 = flat-sequence {
      tunnel: "Start Auto control" -> [w262]
      tunnel: [w263] -> w241
      tunnel: [w261] -> w240
      tunnel: w237 -> [w260]
      tunnel: [w259] -> w236
      tunnel: w235 -> [w259]
      tunnel: w234 -> [w258]
      tunnel: [w257] -> w233
      tunnel: w241 -> [w297]
      tunnel: w240 -> [w301]
      tunnel: [w300] -> w239
      tunnel: [w299] -> w238
      tunnel: w236 -> [w298]
      tunnel: w233 -> [w296]
      frame #0 {
        n135 = case shown="True" w262 {
          tunnel: w260 -> [w266 w279]
          tunnel: [w266 w280] -> w263
          tunnel: [FALSE ("Freq_in Range") w267] -> w261
          tunnel: [w264 w272] -> w257
          tunnel: w258 -> [w264 w272]
          tunnel: "Bypass Freq check" -> [_ w268]
          frame False {
          }
          frame True {
            n136 = property on="Current Frequencuy  (GHz)\n(Mapped)" class="DigNum (strict)"() -> ("Value"=w278:dbl)  [unwired: 2 in, 2 out]
            n137 = Divide(x="Range(MHz)", y=1000.0) -> (x/y=w277:dbl)
            n138 = call "mW_CheckFreq.vi"("Range(GHz)"=w277, "Center Frequency(GHz)"="Center Frequency(GHz)", "Current Frequency"=w278) -> ("Lower"=→"Lower (GHz)":dbl, "Freq_in Range"=w269:bool, "Upper"=→"Upper (GHz)":dbl)  [unwired: 6 in]
            n139 = Or(x=w269, y=w268) -> (x .or. y?=w270:bool)
            n140 = case shown="False" w270 {
              tunnel: [w286 w295] -> w280
              tunnel: w279 -> [w282 w295]
              tunnel: "Center Frequency(GHz)" -> [w285 _]
              tunnel: [FALSE ("Freq_in Range") TRUE ("Freq_in Range")] -> w267
              frame False {
                n141 = call "Check moving.vi"("Motor in"=w282) -> ("IS Move"=w283:bool, "Motor out"=w281:refnum<class "Motor.lvclass">)  [unwired: 8 in, 1 out]
                n142 = case shown="False" w283 {
                  tunnel: [w292 w293] -> w286
                  tunnel: w285 -> [w288 _]
                  tunnel: w281 -> [w287 w293]
                  frame False {
                    n143 = feedback #1() -> (w289:dbl[][])  [unwired: 1 in]
                    n144 = call "conv_FreQ_Pos.vi"("data_in"=w289, "Freq"=w288) -> ("Pos"=w291:dbl, "data_out"=w290:dbl[][])  [unwired: 7 in, 1 out]
                    n145 = feedback-in #1(w290) -> ()
                    n146 = call "Move to possition.vi"("absolute possition(rev)"=w291, "Motor in"=w287) -> ("Motor out"=w292:refnum<class "Motor.lvclass">)  [unwired: 8 in, 1 out]
                  }
                  frame True {
                  }
                }
              }
              frame True {
              }
            }
          }
        }
      }
      frame #1 {
        n147 = case shown="True" w301 {
          tunnel: w298 -> [w303 w312]
          tunnel: [w303 w304] -> w300
          tunnel: [w302 w305] -> w299
          tunnel: w297 -> [_ w308]
          tunnel: w301 -> [_ w307]
          tunnel: w296 -> [w302 w306]
          frame False {
          }
          frame True {
            n148 = call "Has All samples.vi"("error in (no error)"=w306, "Automation in"=w312) -> ("error out"=w311:errorcluster, "Has all samples?"=w309:bool, "Automation out"=w310:refnum<class "Automation.lvclass">)  [unwired: 7 in]
            "Has all samples" <- w309
            n149 = case shown="True" w309 {
              tunnel: w311 -> [w313 w316]
              tunnel: w310 -> [w314 w318]
              tunnel: [w314 w322] -> w304
              tunnel: [w313 w321] -> w305
              tunnel: w308 -> [_ w323]
              tunnel: w307 -> [_ w317]
              frame False {
              }
              frame True {
                n150 = case shown="\"Seek Positive\", Default" "Seek type" {
                  tunnel: [TRUE ("Seek positive polarization?") FALSE ("Seek positive polarization?")] -> w319
                  frame "Seek Positive", Default {
                  }
                  frame "Seek Negative" {
                  }
                }
                n151 = call "Decide next action Rate base_test.vi"("Seek Function"="Seek Function", "error in (no error)"=w316, "Seek?"=w317, "Seek positive polarization?"=w319, "Automation in"=w318) -> ("error out"=w321:errorcluster, "Decision"=w320:T1, "Automation out"=w322:refnum<class "Automation.lvclass">)  [unwired: 1 in, 3 out]
                "Motor Action" <- w320
                n152 = case shown="\"No motion\", Default" w320 {
                  tunnel: [0.0 ("Automatic step size (rev)") w328 w330] -> w324
                  tunnel: "Automatic step size (rev)" -> [_ w329 w330]
                  frame "No motion", Default {
                  }
                  frame "Switch direction" {
                    n153 = Negate(x=w329) -> (-x=w328:dbl)
                    n154 = property on="Automatic step size (rev)" class="DigNum (strict)"("Value"=w328) -> ()  [unwired: 2 in, 2 out]
                  }
                  frame "Keep current direction" {
                  }
                }
                n155 = call "Move.vi"("degrees To move"=w324, "Motor in"=w323) -> ()  [unwired: 8 in, 2 out]
              }
            }
          }
        }
      }
    }
  }
  n156 = while {
    tunnel: w26 -> [w385]
    tunnel: [w384] -> w29
    tunnel: [w387] -> w28
    tunnel: w27 -> [w386]
    tunnel: w3 -> [w381]
    stop <- TRUE stop-if-true
    # "EIP loop"
    n157 = call "Peek or default.vi"("Signaller in"=w381) -> ()  [unwired: 8 in, 3 out]
    n158 = call "mW_EIP_Read.vi"("error in (no error)"=w386, "VISA Refnum in"=w385) -> ("error out"=w387:errorcluster, "Frequency"=w379:dbl, "VISA resource name out"=w384:refnum<visa-resource-name>)  [unwired: 5 in, 1 out]
    "EIP Frequency (GHz)" <- w379
    n159 = property on="Current Frequencuy  (GHz)\n(Mapped)" class="DigNum (strict)"() -> ("Value"=w380:dbl)  [unwired: 2 in, 2 out]
    n160 = Get Date/Time In Seconds() -> (seconds since 1Jan1904=w383:timestamp)
    n161 = call "Create_EIP_waveform_Channel 2.vi"("Mapped"=w380, "time"=w383, "EIP"=w379) -> ("waveform_array"=→"EIPFRQ":waveform(dbl)[])  [unwired: 8 in]
    n162 = Wait (ms)(milliseconds to wait=u32 500) -> ()  [unwired: 1 out]
  }
  n163 = while {
    shift-right: [w408] -> _
    shift-left: TRUE -> [w409]
    tunnel: w33 -> [w407]
    tunnel: w30 -> [w406]
    tunnel: [w405] -> w22
    tunnel: [w404] -> w25
    tunnel: w5 -> [w403]
    tunnel: w23 -> [w402]
    tunnel: [w401] -> w20
    tunnel: [w400] -> w19
    tunnel: w13 -> [w399]
    tunnel: w3 -> [w398]
    tunnel: w11 -> [w396]
    tunnel: w10 -> [w395]
    tunnel: w9 -> [w394]
    tunnel: [w393] -> w8
    tunnel: [w392] -> w7
    tunnel: w4 -> [w391]
    tunnel: w1 -> [w390]
    stop <- w389 stop-if-true
    # "Main Loop"
    n164 = call "Peek or default.vi"("Signaller in"=w398) -> ("error out"=w397:errorcluster, "Has signal?"=w389:bool)  [unwired: 8 in, 1 out]
    n165 = event shown="[14] \"R_lower\": Value Change" {
      selector: _ -> [_ _ _ _ _ _ _ _ _ _ _ _ _ _ _ _ _ _ _]
      dyn-events: _ -> [_ _ _ _ _ _ _ _ _ _ _ _ _ _ _ _ _ _ _]
      timeout: 500 -> [_ _ _ _ _ _ _ _ _ _ _ _ _ _ _ _ _ _ _]
      tunnel: [w424 w505 _ _ _ _ _ _ _ w544 w549 w562 w573 w586 _ _ w614 w624 w636] -> w405
      tunnel: [w433 w503 _ _ _ _ _ _ _ _ w551 w570 _ w582 w587 w599 w621 w630 w639] -> w400
      tunnel: w407 -> [w435 w503 _ _ _ _ _ _ _ _ w551 w570 _ w582 w587 w599 w621 w630 w639]
      tunnel: w406 -> [w436 w502 _ _ _ _ _ _ _ w546 w552 w569 _ w581 w588 w600 w622 w629 w640]
      tunnel: [w431 w502 _ _ _ _ _ _ _ w546 w552 w569 _ w581 w588 w600 w622 w629 w640] -> w404
      tunnel: w403 -> [w430 w507 _ _ _ _ _ _ _ w548 w550 w568 w577 _ _ _ w620 w626 w637]
      tunnel: w402 -> [w429 w504 _ _ _ _ _ _ _ w547 w549 w567 _ _ _ _ w619 w627 w638]
      tunnel: [w425 w507 _ _ _ _ _ _ _ w543 w550 w560 w571 _ _ _ w612 w625 w635] -> w401
      tunnel: w399 -> [_ _ _ _ _ _ w530 _ _ _ _ _ _ _ _ _ _ _ _]
      tunnel: w398 -> [_ _ _ _ _ _ _ _ w540 _ _ _ _ _ _ _ _ _ _]
      tunnel: w397 -> [_ _ _ _ _ _ _ _ w539 _ _ _ _ _ _ _ _ _ _]
      tunnel: w396 -> [w413 _ _ _ _ _ _ _ _ _ _ _ _ _ _ _ _ _ _]
      tunnel: w395 -> [w421 w506 _ _ _ _ _ _ _ _ _ _ _ _ _ _ _ _ _]
      tunnel: w394 -> [w419 w505 _ _ _ _ _ _ _ _ _ _ _ _ _ _ _ _ _]
      tunnel: [w417 w506 _ _ _ _ _ _ _ _ _ _ _ _ _ _ _ _ _] -> w393
      tunnel: [w415 w504 _ _ _ _ _ _ _ _ _ _ _ _ _ _ _ _ _] -> w392
      tunnel: w391 -> [w411 _ _ _ _ _ _ _ _ _ _ _ _ _ _ _ _ _ _]
      tunnel: w390 -> [_ _ _ _ _ _ _ _ _ _ _ _ _ _ _ _ _ _ _]
      event Timeout {
        n166 = event-data() -> ()  [unwired: 1 in, 3 out]
        n167 = flat-sequence {
          tunnel: w435 -> [w467]
          tunnel: [w466] -> w438
          tunnel: w436 -> [w463]
          tunnel: [w462] -> w434
          tunnel: w430 -> [w455]
          tunnel: w429 -> [w454]
          tunnel: [w447] -> w428
          tunnel: [w449] -> w423
          tunnel: [w442] -> w422
          tunnel: w421 -> [w442]
          tunnel: [w441] -> w420
          tunnel: w419 -> [w441]
          tunnel: w413 -> [w440]
          tunnel: [w440] -> w414
          tunnel: [w439] -> _
          tunnel: [w439] -> w412
          tunnel: w411 -> [w439]
          tunnel: w438 -> [w482]
          tunnel: [w482] -> w437
          tunnel: w434 -> [w481]
          tunnel: [w481] -> w432
          tunnel: w428 -> [w480]
          tunnel: [w480] -> w427
          tunnel: [w479] -> w426
          tunnel: w423 -> [w479]
          tunnel: w422 -> [w475]
          tunnel: w420 -> [w474]
          tunnel: [w473] -> w418
          tunnel: [w472] -> w416
          tunnel: w414 -> [w470]
          tunnel: w412 -> [w469]
          tunnel: [w496] -> w424
          tunnel: [w499] -> w433
          tunnel: w437 -> [w499]
          tunnel: w432 -> [w498]
          tunnel: [w498] -> w431
          tunnel: w427 -> [w496]
          tunnel: w426 -> [w497]
          tunnel: [w497] -> w425
          tunnel: [w495] -> w417
          tunnel: w418 -> [w495]
          tunnel: [w494] -> w415
          tunnel: w416 -> [w494]
          frame #0 {
            n168 = call "Check moving.vi"("error in (no error)"=w454, "Motor in"=w455) -> ("error out"=w458:errorcluster, "IS Move"=→"Motor Running":bool, "Motor out"=w453:refnum<class "Motor.lvclass">)  [unwired: 7 in]
            n169 = call "Get Possition.vi"("error in (no error)"=w458, "Motor in"=w453) -> ("error out"=w457:errorcluster, "Revolutions"=w446:dbl, "Motor out"=w452:refnum<class "Motor.lvclass">)  [unwired: 7 in]
            "Current motor possition (Revolutions)" <- w446
            "Current possition (rev)" <- w446
            n170 = call "mWADC_AVG_out.vi"("error out"=w463, "reference out"=w467) -> ("error out 2"=w462:errorcluster, "ADC_avg_out"=w464:i32, "VISA resource name out"=w466:refnum<visa-resource-name>)  [unwired: 7 in]
            "ADC Count" <- w464
            "ADC Count" <- w464
            n171 = call "check limits.vi"("error in (no error)"=w457, "Motor in"=w452) -> ("error out"=w456:errorcluster, "Negetive_L"=→"CW":bool, "Positive_L"=→"CCW":bool, "Motor out"=w451:refnum<class "Motor.lvclass">)  [unwired: 6 in]
            n172 = call "adcTOrev.vi"("ADC count"=w464) -> ("Estimated Possition"=→"Estimated Possition":dbl)  [unwired: 10 in]
            n173 = call "Get Alarm.vi"("error in (no error)"=w456, "Motor in"=w451) -> ("error out"=w448:errorcluster, "Motor alarm?"=w450:bool, "Motor out"=w449:refnum<class "Motor.lvclass">)  [unwired: 6 in, 1 out]
            "Motor alarm" <- w450
            n174 = property on="Motor alarm" class="Bool (strict)"("Blinking"=w450) -> ()  [unwired: 2 in, 2 out]
            n175 = feedback #2() -> (w444:dbl[][])  [unwired: 1 in]
            n176 = call "conv_Pos_Fre.vi"("data_in"=w444, "error in"=w448, "Pos"=w446) -> ("error out"=w447:errorcluster, "FreQ"=→"Current Frequencuy  (GHz)\n(Mapped)":dbl, "data_out"=w445:dbl[][])  [unwired: 6 in]
            n177 = feedback-in #2(w445) -> ()
          }
          frame #1 {
            n178 = call "mW_EIOTemp_check.vi"("Temp Gradients"=w469, "EIO temp"=w470) -> ("Temp alarms"=w471:bool)  [unwired: 9 in]
            "Temp alarms" <- w471
            n179 = case shown="False" w471 {
              tunnel: [T2."Disabled and Grayed Out" ("Disabled") T2."Enabled" ("Disabled")] -> w468
              frame False {
                n180 = property on="Recovery sequence" class="Str"("Value"="") -> ()  [unwired: 2 in, 2 out]
              }
              frame True {
              }
            }
            n181 = And(x=w471, y="Warning Sound") -> (x .and. y?=w476:bool)
            n182 = property on="EIO Temp" class="Str"("Blinking"=w471) -> ()  [unwired: 2 in, 2 out]
            n183 = property on="EIO Temp" class="Str"("Visible"=w471) -> ()  [unwired: 2 in, 2 out]
            n184 = case shown="False" w476 {
              tunnel: w475 -> [w489 w493]
              tunnel: w474 -> [w487 w492]
              tunnel: [w488 w491] -> w473
              tunnel: [w486 w490] -> w472
              frame False {
                n185 = call <vilib>:"Sound Output Stop.vi"("error in (no error)"=w487, "task ID"=w489) -> ("error out"=w486:errorcluster, "task ID out"=w488:T3)  [unwired: 8 in]
              }
              frame True {
                n186 = call "Play Warning.vi"("error in (no error)"=w492, "task ID"=w493) -> ("error out"=w490:errorcluster, "task ID 2"=w491:T3)  [unwired: 8 in]
              }
            }
            n187 = property on="Recovery" class="Bool (strict)"("DisabledEnum"=w468) -> ()  [unwired: 2 in, 2 out]
            "EIO Temp" <- "EIO Temperature is low\nCheck the power supply for warnings  " ("EIP Lost")
          }
          frame #2 {
          }
        }
      }
      event "Seek type": Value Change {
        n188 = event-data() -> ()  [unwired: 1 in, 6 out]
        n189 = property on="Seek type" class="RadioBtnsControl (strict)"() -> ("Value"=w501:enum32{"Seek Positive", "Seek Negative"})  [unwired: 2 in, 2 out]
        n190 = case shown="\"Seek Positive\", Default" w501 {
          tunnel: [140.2 ("Center Frequency(GHz)") 140.5 ("Center Frequency(GHz)")] -> w500
          frame "Seek Positive", Default {
          }
          frame "Seek Negative" {
          }
        }
        n191 = property on="Center Frequency(GHz)" class="DigNum (strict)"("Value"=w500) -> ()  [unwired: 2 in, 2 out]
      }
      event "Reset the counter": Value Change {
        n192 = event-data() -> ()  [unwired: 1 in, 6 out]
      }
      event "Recovery": Value Change {
        n193 = event-data() -> ()  [unwired: 1 in, 6 out]
        n194 = property on="Start Recovery" class="Bool (strict)"("Value"=TRUE ("Start Recovery")) -> ()  [unwired: 2 in, 2 out]
      }
      event "Start calibration": Value Change {
        n195 = event-data() -> ()  [unwired: 1 in, 6 out]
        n196 = property on="Motor Running" class="Bool (strict)"() -> ("Value"=w512:bool)  [unwired: 2 in, 2 out]
        n197 = property on="Start Auto control" class="Bool (strict)"() -> ("Value"=w513:bool)  [unwired: 2 in, 2 out]
        n198 = And(x=w512, y=w513) -> (x .and. y?=w514:bool)
        n199 = case shown="False" w514 {
          tunnel: [w515 FALSE ("Calibration run flag")] -> w511
          frame False {
            n200 = call "Display Message to User2"() -> ("Yes"=w516:bool)  [unwired: 10 in, 1 out]
            n201 = case shown="True" w516 {
              tunnel: [FALSE ("Calibration run flag") TRUE ("Calibration run flag")] -> w515
              frame False {
              }
              frame True {
              }
            }
          }
          frame True {
            n202 = call "Display Message to User"() -> ()  [unwired: 10 in, 2 out]
          }
        }
        "Calibration run flag" <- w511
        n203 = property on="Recording" class="Bool (strict)"("Blinking"=w511) -> ()  [unwired: 2 in, 2 out]
      }
      event "Stop calibration": Value Change {
        n204 = event-data() -> ()  [unwired: 1 in, 6 out]
        n205 = property on="stop motor" class="Bool (strict)"("Val(Sgnl)"=FALSE ("Value (Signaling)")) -> ()  [unwired: 2 in, 2 out]
        n206 = property on="Recording" class="Bool (strict)"("Blinking"=FALSE) -> ()  [unwired: 2 in, 2 out]
        n207 = property on="Calibration run flag" class="Bool (strict)"("Value"=FALSE ("Calibration run flag")) -> ()  [unwired: 2 in, 2 out]
      }
      event "Launch simulation": Value Change {
        n208 = event-data() -> ()  [unwired: 1 in, 6 out]
        n209 = invoke class="VI (strict)" method="FP.Open"(reference=w530) -> (reference out=w524:refnum<vi>, error out=w523:errorcluster)  [unwired: 4 in, 3 out]
        n210 = property class="VI Interface Type 0"(reference=w524, error in=w523) -> (reference out=w529:refnum<vi>, error out=w528:errorcluster, "Exec.State"=w527:T4)
        n211 = Equal?(x=w527, y=T4."Idle" ("Execution:State")) -> (x = y?=w525:bool)
        n212 = case shown="True" w525 {
          tunnel: w529 -> [_ w534]
          tunnel: w528 -> [w531 w533]
          tunnel: [w531 w532] -> _
          frame False {
          }
          frame True {
            n213 = invoke class="VI (strict)" method="Run VI"(reference=w534, error in=w533, "Wait until done"=FALSE ("Wait Until Done"), "Auto Dispose Ref"=TRUE ("Auto Dispose Reference")) -> (error out=w532:errorcluster)  [unwired: 1 in, 4 out]
          }
        }
      }
      event "Calibration panel": Value Change {
        n214 = event-data() -> ()  [unwired: 1 in, 6 out]
        n215 = property on="Calibration panel" class="TabCtl (strict)"("Visible"="Calibration panel") -> ()  [unwired: 2 in, 2 out]
        n216 = call "Close thermocouple VI.vi"() -> ()  [unwired: 11 in, 1 out]
      }
      event "stop VI": Value Change {
        (unwired) TRUE ("stop")
        n217 = event-data() -> ()  [unwired: 1 in, 3 out]
        n218 = property on="Polarization data source" class="RadioBtnsControl (strict)"("DisabledEnum"=T2."Enabled" ("Disabled")) -> ()  [unwired: 2 in, 2 out]
        n219 = call "Signal.vi"("error in (no error)"=w539, "Signaller in"=w540) -> ()  [unwired: 8 in, 2 out]
      }
      event "stop motor": Value Change {
        n220 = event-data() -> ()  [unwired: 1 in, 5 out]
        n221 = call "Stop.vi"("error in (no error)"=w547, "Motor in"=w548) -> ("error out"=w545:errorcluster, "Motor out"=w543:refnum<class "Motor.lvclass">)  [unwired: 8 in]
        n222 = call "Get Possition.vi"("error in (no error)"=w545, "Motor in"=w543) -> ("error out"=w544:errorcluster, "Revolutions"=w542:dbl)  [unwired: 7 in, 1 out]
        n223 = property on="Set possition (rev)" class="DigNum (strict)"("Value"=w542) -> ()  [unwired: 2 in, 2 out]
        n224 = property on="Recovery loop stop" class="Bool (strict)"("Value"=TRUE ("Recovery loop stop")) -> ()  [unwired: 2 in, 2 out]
      }
      event "cal_para": Value Change {
        n225 = event-data() -> ()  [unwired: 1 in, 5 out]
        n226 = property on="Upper  possition" class="DigNum (strict)"() -> ("Value"=w555:dbl)  [unwired: 2 in, 2 out]
        n227 = property on="Lower  possition" class="DigNum (strict)"() -> ("Value"=w556:dbl)  [unwired: 2 in, 2 out]
        n228 = property on="Lower Frequency" class="DigNum (strict)"() -> ("Value"=w557:dbl)  [unwired: 2 in, 2 out]
        n229 = property on="Upper Frequecy" class="DigNum (strict)"() -> ("Value"=w558:dbl)  [unwired: 2 in, 2 out]
        n230 = formula code="m=(y2-y1)/(x2-x1);\nc=y2-m*x2;"("x1"=w556, "y1"=w557, "x2"=w555, "y2"=w558) -> ("m"=→"New Slope":dbl, "c"=→"New Intercept":dbl)
      }
      event "CW": Value Change {
        n231 = event-data() -> ()  [unwired: 1 in, 6 out]
        n232 = local read "Degrees"() -> (w565:dbl)
        n233 = Divide(x=w565, y=360.0) -> (x/y=w564:dbl)
        n234 = call "Move.vi"("error in (no error)"=w567, "degrees To move"=w564, "Motor in"=w568) -> ("error out"=w563:errorcluster, "Motor out"=w561:refnum<class "Motor.lvclass">)  [unwired: 7 in]
        n235 = call "Get Possition.vi"("error in (no error)"=w563, "Motor in"=w561) -> ("error out"=w562:errorcluster, "Revolutions"=w559:dbl, "Motor out"=w560:refnum<class "Motor.lvclass">)  [unwired: 7 in]
        n236 = property on="Set possition (rev)" class="DigNum (strict)"("Value"=w559) -> ()  [unwired: 2 in, 2 out]
      }
      event "Set_motor": Value Change {
        n237 = event-data() -> ()  [unwired: 1 in, 6 out]
        n238 = call "mWmotor_set_motor_para.vi"("configuration file path"="File Path Control") -> ("Intercept"=→"Intercept":dbl, "Slope"=→"Slope":dbl, "Speed"=w576:string)  [unwired: 8 in]
        n239 = call "SetSpeed.vi"("Speed"=w576, "Motor in"=w577) -> ("error out"=w574:errorcluster, "Motor out"=w575:refnum<class "Motor.lvclass">)  [unwired: 8 in]
        n240 = call "Get Speed.vi"("error in (no error)"=w574, "Motor in"=w575) -> ("error out"=w573:errorcluster, "Speed"=→"Speed  (rev/s)":dbl, "Motor out"=w571:refnum<class "Motor.lvclass">)  [unwired: 7 in]
      }
      event "Use_para": Value Change {
        n241 = event-data() -> ()  [unwired: 1 in, 6 out]
        n242 = property on="File Path Control" class="Path"() -> ("Value"=w585:path)  [unwired: 2 in, 2 out]
        n243 = property on="New Slope" class="DigNum (strict)"() -> ("Value"=w583:dbl)  [unwired: 2 in, 2 out]
        n244 = property on="New Intercept" class="DigNum (strict)"() -> ("Value"=w584:dbl)  [unwired: 2 in, 2 out]
        n245 = property on="Intercept" class="DigNum (strict)"("Value"=w584) -> ()  [unwired: 2 in, 2 out]
        n246 = property on="Slope" class="DigNum (strict)"("Value"=w583) -> ()  [unwired: 2 in, 2 out]
        n247 = call "mWmotor_write_fitparameter.vi"("Intercept"=w584, "Slope"=w583, "configuration file path"=w585) -> ("error out"=w586:errorcluster)  [unwired: 8 in]
      }
      event "R_lower": Value Change {
        w592 = 100
        n248 = event-data() -> ()  [unwired: 1 in, 6 out]
        n249 = property on="EIP Frequency (GHz)" class="DigNum (strict)"() -> ("Value"=w590:dbl)  [unwired: 2 in, 2 out]
        n250 = property on="Current possition (rev)" class="DigNum (strict)"() -> ("Value"=→"Lower  possition":dbl)  [unwired: 2 in, 2 out]
        n251 = for {
          N: w592 -> [_]
          shift-right: [w597] -> w593
          shift-left: 0.0 ("y") -> [w598]
          tunnel: w590 -> [w596]
          n252 = Add(x=w598, y=w596) -> (x+y=w597:dbl)
        }
        n253 = Divide(x=w593, y=w592) -> (x/y=→"Lower Frequency":dbl)
        n254 = Wait (ms)(milliseconds to wait=u32 100) -> ()  [unwired: 1 out]
      }
      event "R_upper": Value Change {
        w605 = 100
        n255 = event-data() -> ()  [unwired: 1 in, 6 out]
        n256 = property on="EIP Frequency (GHz)" class="DigNum (strict)"() -> ("Value"=w602:dbl)  [unwired: 2 in, 2 out]
        n257 = property on="Current possition (rev)" class="DigNum (strict)"() -> ("Value"=→"Upper  possition":dbl)  [unwired: 2 in, 2 out]
        n258 = for {
          N: w605 -> [_]
          shift-right: [w609] -> w606
          shift-left: 0.0 ("y") -> [w610]
          tunnel: w602 -> [w608]
          n259 = Add(x=w610, y=w608) -> (x+y=w609:dbl)
        }
        n260 = Divide(x=w606, y=w605) -> (x/y=→"Upper Frequecy":dbl)
        n261 = Wait (ms)(milliseconds to wait=u32 100) -> ()  [unwired: 1 out]
      }
      event "CCW": Value Change {
        n262 = event-data() -> ()  [unwired: 1 in, 3 out]
        n263 = Negate(x="Degrees") -> (-x=w617:dbl)
        n264 = Divide(x=w617, y=360.0) -> (x/y=w618:dbl)
        n265 = call "Move.vi"("error in (no error)"=w619, "degrees To move"=w618, "Motor in"=w620) -> ("error out"=w615:errorcluster, "Motor out"=w613:refnum<class "Motor.lvclass">)  [unwired: 7 in]
        n266 = call "Get Possition.vi"("error in (no error)"=w615, "Motor in"=w613) -> ("error out"=w614:errorcluster, "Revolutions"=w611:dbl, "Motor out"=w612:refnum<class "Motor.lvclass">)  [unwired: 7 in]
        n267 = property on="Set possition (rev)" class="DigNum (strict)"("Value"=w611) -> ()  [unwired: 2 in, 2 out]
      }
      event "Set possition (rev)": Value Change {
        n268 = event-data() -> ()  [unwired: 1 in, 3 out]
        n269 = call "Move to possition.vi"("error in (no error)"=w627, "absolute possition(rev)"="Set possition (rev)", "Motor in"=w626) -> ("error out"=w624:errorcluster, "Motor out"=w625:refnum<class "Motor.lvclass">)  [unwired: 7 in]
      }
      event "Move to frequecy": Value Change {
        n270 = event-data() -> ()  [unwired: 1 in, 3 out]
        n271 = feedback #3() -> (w632:dbl[][])  [unwired: 1 in]
        n272 = call "conv_FreQ_Pos.vi"("data_in"=w632, "Freq"="Set Freq (GHz)") -> ("Pos"=w634:dbl, "data_out"=w633:dbl[][])  [unwired: 7 in, 1 out]
        n273 = feedback-in #3(w633) -> ()
        n274 = property on="Center Frequency(GHz)" class="DigNum (strict)"("Value"="Set Freq (GHz)") -> ()  [unwired: 2 in, 2 out]
        n275 = call "Move to possition.vi"("error in (no error)"=w638, "absolute possition(rev)"=w634, "Motor in"=w637) -> ("error out"=w636:errorcluster, "Motor out"=w635:refnum<class "Motor.lvclass">)  [unwired: 7 in]
      }
    }
    n276 = Not(x=w409) -> (.not. x?=w408:bool)
    "Loop Running" <- w409
  }
  n277 = call "Clear sound buffer.vi"("error in (no error)"=w7, "task ID"=w8) -> ("error out"=w6:errorcluster)  [unwired: 9 in]
  n278 = VISA Close(VISA resource name=w29, error in (no error)=w28) -> (error out=w24:errorcluster)
  n279 = VISA Close(VISA resource name=w19, error in (no error)=w25) -> (error out=w32:errorcluster)
  n280 = call "Close Port.vi"("error in (no error)"=w22, "Motor in"=w20) -> ("error out"=w21:errorcluster)  [unwired: 9 in]
  n281 = Merge Errors(w6, w21, w32, w24, w14) -> (→"error out":errorcluster)
